vi "Get System Exit Event Registration.vi"(11 "Mediated Actor in":refnum<class "Mediated Actor.lvclass">) -> (2 "System Exit Registration":refnum<event-registration>, 3 "Mediated Actor out":refnum<class "Mediated Actor.lvclass">)   [LabVIEW 2016, in "Stream Mediator.lvlib" / "Mediated Actor.lvclass"]
uses:
  <userlib>/Composed Systems/Stream/Mediator/Classes/Mediated Actor/Mediated Actor.lvclass
  <userlib>/Composed Systems/Stream/Mediator/Classes/Message Interface/Message Interface.lvclass
  <userlib>/Composed Systems/Stream/Mediator/Classes/Mediated Actor/Mediated Actor.lvclass/Mediated Actor.ctl
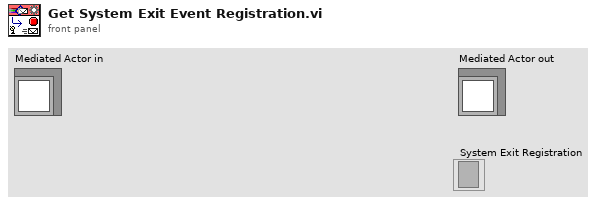
[diagram p1: front panel]
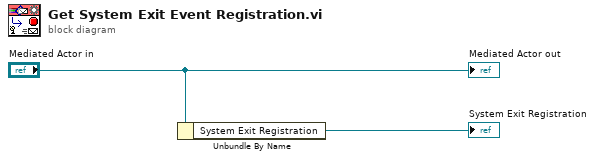
[diagram p0: block diagram]
diagram:
  n1 = Unbundle By Name("Mediated Actor in") -> ("System Exit Registration"=→"System Exit Registration":refnum<event-registration>)
  "Mediated Actor out" <- "Mediated Actor in"
